vi "Target Colour v2.vi"() -> (3 "Threshold Image":T1(plugin-control))   [LabVIEW 2013]
uses:
  <vilib>/Rock Robotics/WPI/Camera/WPI_CameraSettings Read MJPG.ctl
  <vilib>/Rock Robotics/WPI/Camera/WPI_CameraImageSize.ctl
  <vilib>/vision/NI_Vision_Development_Module.lvlib
panel:
  in  "Camera view angle":dbl=33.7 format="%#_13g"
  out "Distance (cm)":dbl=163.65164688042847
  out "Number of Particles":i32=1
  in  "Blue or Luminance":cluster{i32, i32}(slide)={130, 255} scale=0.0..255.0
  in  "Green or Saturation":cluster{i32, i32}(slide)={0, 255} scale=0.0..255.0
  in  "Threshold Color Mode":enum32{"RGB", "HSL"}(radio)=enum."HSL"
  in  "Red or Hue":cluster{i32, i32}(slide)={53, 255} scale=0.0..255.0
  in  "stop":bool
  in  "Camera Settings":T2={"fps"=15, "compression"=5, "Image Size"=enum."320x240"}
  in  "Camera IP":string="10.40.1.11"
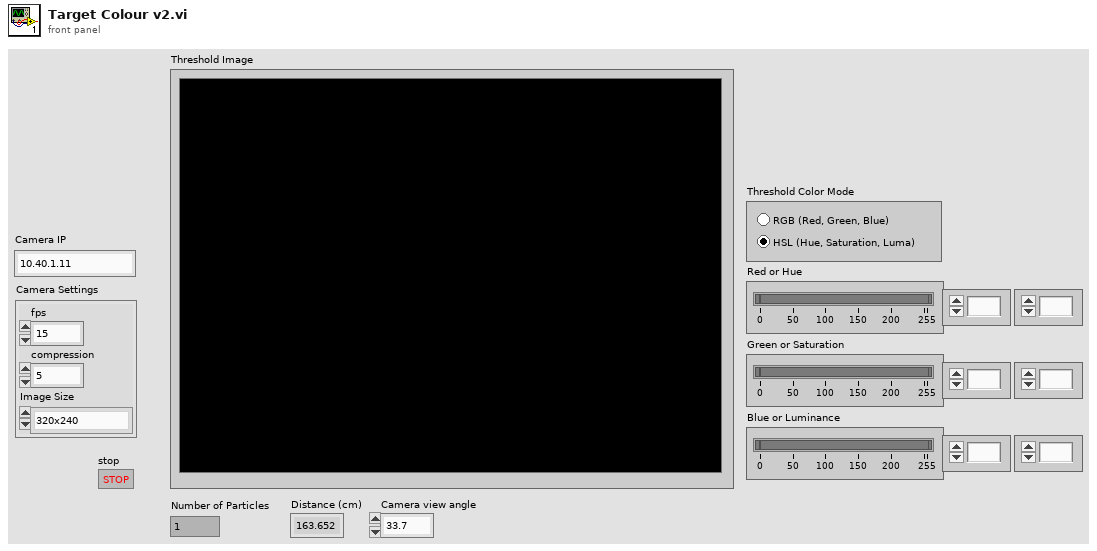
[diagram p1: front panel]
types:
  T1 = typedef "IMAQ Image.ctl" = refnum<image>
  T2 = typedef "WPI_CameraSettings Read MJPG.ctl" = cluster{"fps":i32, "compression":i32, "Image Size":T3}
  T3 = typedef "WPI_CameraImageSize.ctl" = enum16{"640x480", "320x240", "160x120"}
  T4 = typedef "Image Type" = u32
  T5 = typedef "IMAQ Rectangle" = cluster{"Left":i32, "Top":i32, "Right":i32, "Bottom":i32, "Rotation":dbl}
  T6 = typedef "ROI Descriptor" = cluster{"Global Rectangle":i32[], "Contours":cluster{"ID":enum32{"External", "Internal"}, "Type":u32, "Coordinates":i32[]}[]}
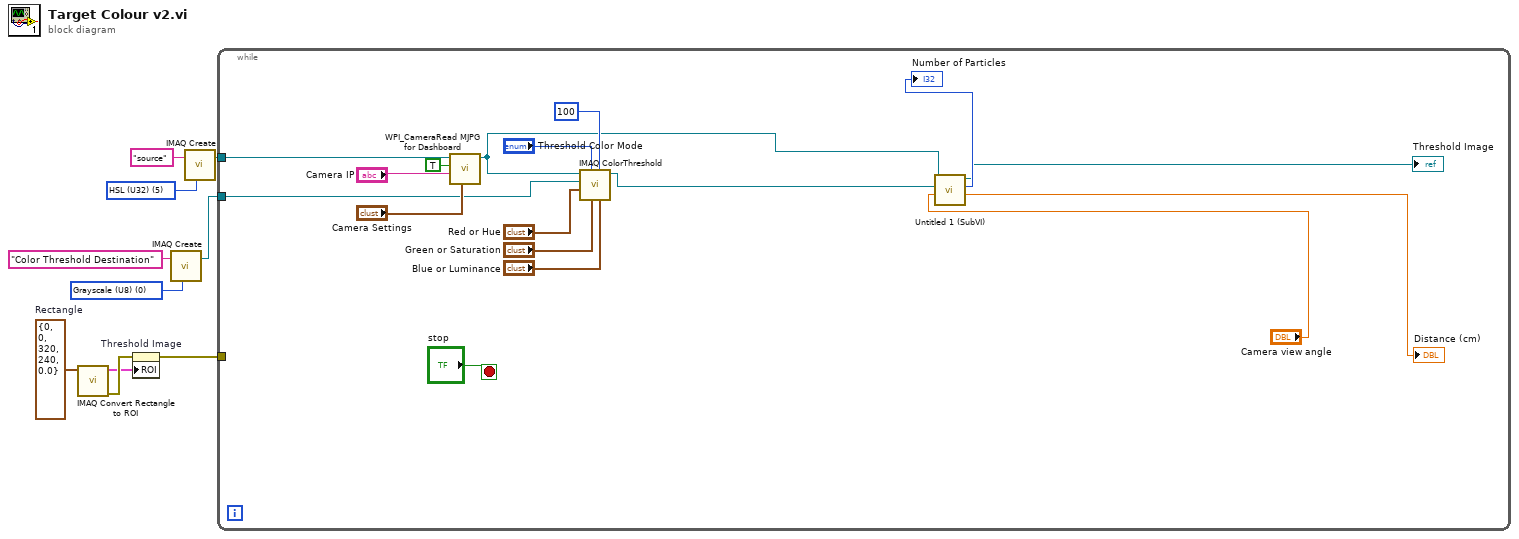
[diagram p0: block diagram]
diagram:
  w4 = T4 0 items=["Grayscale (U8)", "Grayscale (I16)", "Grayscale (SGL)", "Complex (CSG)", "RGB (U32)", "HSL (U32)", "RGB (U64)", "Grayscale (U16)"] ("Image Type")
  w7 = T5 {"Left"=0, "Top"=0, "Right"=320, "Bottom"=240, "Rotation"=0.0}  # Rectangle
  w8 = T4 5 items=["Grayscale (U8)", "Grayscale (I16)", "Grayscale (SGL)", "Complex (CSG)", "RGB (U32)", "HSL (U32)", "RGB (U64)", "Grayscale (U16)"] ("Image Type")
  n1 = call "IMAQ Convert Rectangle to ROI"("Rectangle"=w7) -> ("error out"=w6:errorcluster, "ROI Descriptor"=w5:T6)  [unwired: 8 in]
  n2 = property on="Threshold Image" class="ImageControl"(error in=w6, "ROI"=w5) -> (error out=w1:errorcluster)  [unwired: 1 in, 1 out]
  n3 = call "IMAQ Create"("Image Name"="Color Threshold Destination", "Image Type"=w4) -> ("New Image"=w3:T1)  [unwired: 3 in, 1 out]
  n4 = call "IMAQ Create"("Image Name"="source", "Image Type"=w8) -> ("New Image"=w9:T1)  [unwired: 3 in, 1 out]
  n5 = while {
    tunnel: w9 -> [w23]
    tunnel: w3 -> [w18]
    tunnel: w1 -> [_]
    stop <- "stop" stop-if-true
    n6 = call <vilib>:"WPI_CameraRead MJPG for Dashboard.vi"("Camera Settings"="Camera Settings", "Camera IP"="Camera IP", "Enable"=TRUE, "Refnum in"=w23) -> ("Refnum out"=w14:T1)  [unwired: 4 in, 3 out]
    n7 = call "IMAQ ColorThreshold"("Blue or Luma or Val or Inten Range"="Blue or Luminance", "Replace Value"=100, "Green or Sat Range"="Green or Saturation", "Color Mode"="Threshold Color Mode", "Red or Hue Range"="Red or Hue", "Image Dst"=w18, "Image Src"=w14) -> ("Image Dst Out"=w16:T1)  [unwired: 3 in, 1 out]
    n8 = call "Untitled 1 (SubVI).vi"("Camera view angle"="Camera view angle", "Image Dst Out"=w16, "Refnum in"=w14) -> ("Distance (cm)"=→"Distance (cm)":dbl, "Number of Particles"=→"Number of Particles":i32, "Refnum out"=→"Threshold Image":T1)  [unwired: 6 in]
  }
